vi "Import File - Rx XML.vi"(6 "Root Node":refnum<k24>, 8 "error in (no error)":errorcluster) -> (0 "error out":errorcluster, 5 "Rx Packets":T1 {"Rx Packet Data"."Endianness" items=["big-endian"=0, "little-endian"=2]})   [LabVIEW 2016, in "UDP-Custom-Device System Explorer.lvlib"]
uses:
  UDP-Custom-Device System Explorer.lvlib
  System.Xml
  Types/XML - New/ImpExp - Rx Packets Data.ctl
  <vilib>/NI Veristand/Custom Device API/Custom Device Item Info.ctl
  Types/XML - New/ImpExp - Rx Packet Data.ctl
  Shared/Types/Shared - Channel Data Type.ctl
  Shared/Types/Shared - Buffered.PacketInfo.ctl
  Shared/Types/Shared - Pointer Encoding.ctl
  <vilib>/NI VeriStand/Custom Device API/Custom Device API.lvlib
  Shared/UDP-Custom-Device Shared.lvlib
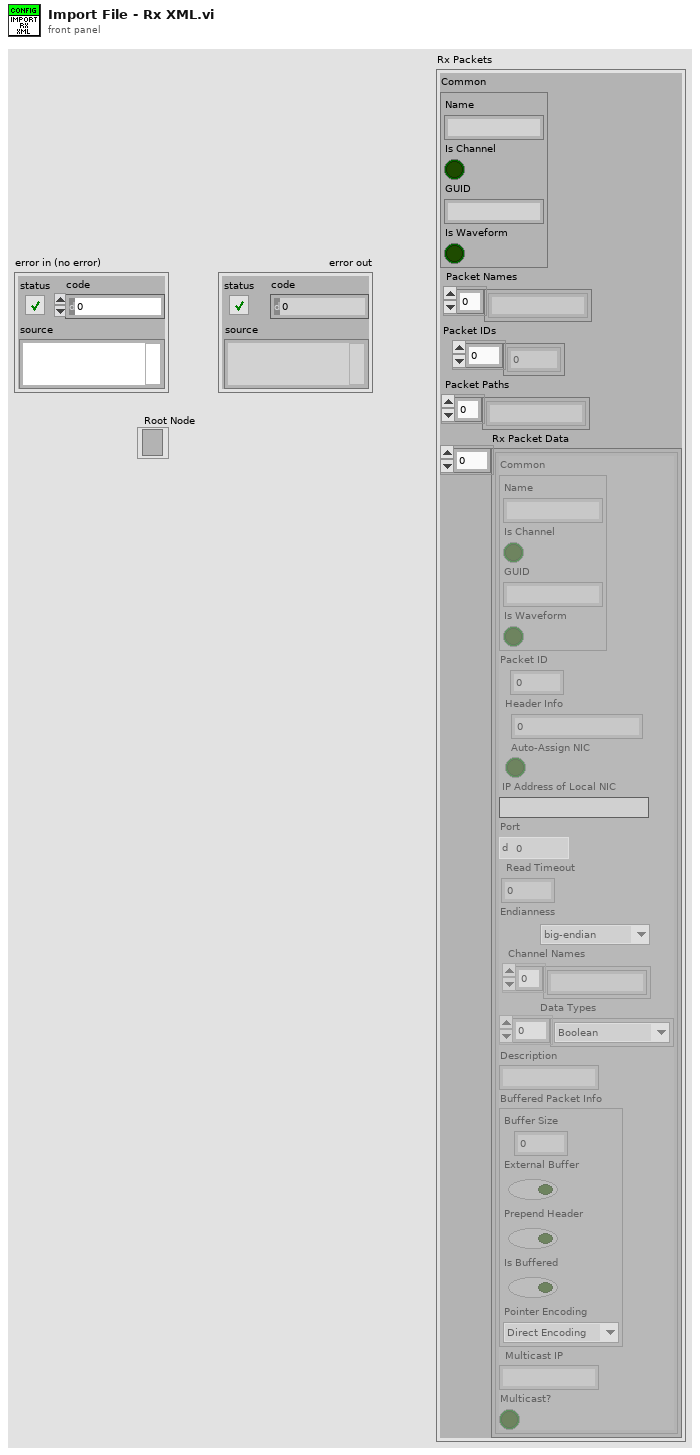
[diagram p1: front panel]
types:
  T1 = typedef "UDP-Custom-Device System Explorer.lvlib/ImpExp - Rx Packets Data.ctl" = cluster{"Common":T2, "Packet Names":string[], "Packet IDs":i32[], "Packet Paths":string[], "Rx Packet Data":T3[]}
  T2 = typedef "Custom Device API.lvlib/Custom Device Item Info.ctl" = cluster{"Name":string, "Is Channel":bool, "GUID":string, "Is Waveform":bool}
  T3 = typedef "UDP-Custom-Device System Explorer.lvlib/ImpExp - Rx Packet Data.ctl" = cluster{"Common":T2, "Packet ID":i32, "Header Info":u32, "Auto-Assign NIC":bool, "IP Address of Local NIC":string, "Port":u16, "Read Timeout":i32, "Endianness":u16, "Channel Names":string[], "Data Types":T4[], "Description":string, "Buffered Packet Info":T5, "Multicast IP":string, "Multicast?":bool}
  T4 = typedef "UDP-Custom-Device Shared.lvlib/Shared - Channel Data Type.ctl" = enum16{"Boolean", "Single", "Double", "I8", "I16", "I32", "I64", "U8", "U16", "U32", "U64"}
  T5 = typedef "UDP-Custom-Device Shared.lvlib/Shared - Buffered.PacketInfo.ctl" = cluster{"Buffer Size":i32, "External Buffer":bool, "Prepend Header":bool, "Is Buffered":bool, "Pointer Encoding":T6}
  T6 = typedef "UDP-Custom-Device Shared.lvlib/Shared - Pointer Encoding.ctl" = enum16{"Direct Encoding", "Conversion Encoding"}
  T7 = typedef "UDP-Custom-Device System Explorer.lvlib/ImpExp - Packet Headers.ctl" = cluster{"Packet Name":string, "Packet ID":string, "Packet Path":string}
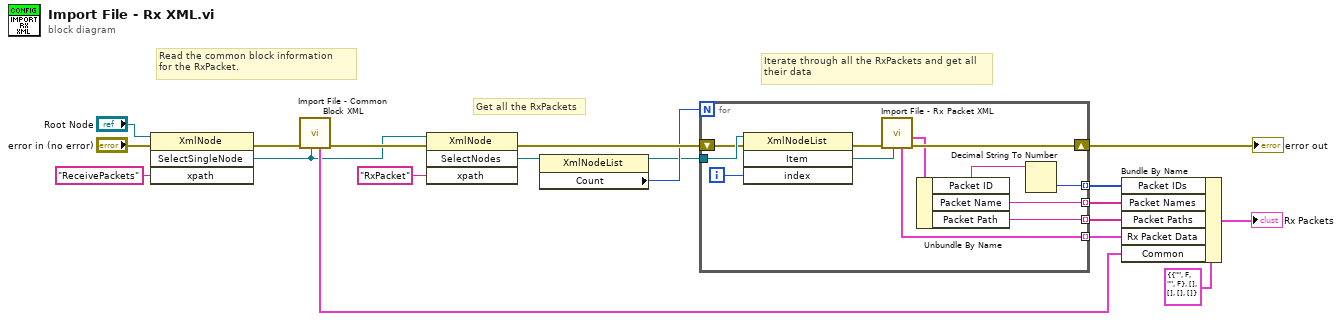
[diagram p0: block diagram]
diagram:
  # "Iterate through all the RxPackets and get all\ntheir data"
  # "Get all the RxPackets"
  # "Read the common block information\nfor the RxPacket."
  n1 = invoke class="XmlNode" method="SelectSingleNode"(reference="Root Node", error in="error in (no error)", "xpath"="ReceivePackets") -> (error out=w16:errorcluster, "SelectSingleNode"=w9:refnum<k24>)  [unwired: 1 in, 2 out]
  n2 = call "Import File - Common Block XML.vi"("Root Node"=w9, "error in (no error)"=w16) -> ("error out"=w11:errorcluster, "Common"=w14:T2)  [unwired: 8 in]
  n3 = invoke class="XmlNode" method="SelectNodes"(reference=w9, error in=w11, "xpath"="RxPacket") -> (error out=w10:errorcluster, "SelectNodes"=w7:refnum<k24>)  [unwired: 1 in, 2 out]
  n4 = property class="XmlNodeList"(reference=w7) -> (reference out=w5:refnum<k24>, "Count"=w6:i32)  [unwired: 1 in, 1 out]
  n5 = for {
    N: w6 -> [_]
    shift-right: [w27] -> w13
    shift-left: w10 -> [w30]
    tunnel: w5 -> [w31]
    tunnel: [w25] -> w4 mode=indexing
    tunnel: [w22] -> w3 mode=indexing
    tunnel: [w21] -> w2 mode=indexing
    tunnel: [w20] -> w1 mode=indexing
    i -> [w29]
    n6 = invoke class="XmlNodeList" method="Item"(reference=w31, error in=w30, "index"=w29) -> (error out=w28:errorcluster, "Item"=w26:refnum<k24>)  [unwired: 1 in, 2 out]
    n7 = call "Import File - Rx Packet XML.vi"("Root Node"=w26, "error in (no error)"=w28) -> ("error out"=w27:errorcluster, "Rx Header Data"=w24:T7, "Rx Packet"=w25:T3)  [unwired: 7 in]
    n8 = Unbundle By Name(w24) -> ("Packet ID"=w23:string, "Packet Name"=w21:string, "Packet Path"=w20:string)
    n9 = Decimal String To Number(string=w23) -> (number=w22:i32)  [unwired: 2 in, 1 out]
  }
  "error out" <- w13
  n10 = Bundle By Name(cluster=T1 {"Common"={"Name"="", "Is Channel"=FALSE, "GUID"="", "Is Waveform"=FALSE}, "Packet Names"=[], "Packet IDs"=[], "Packet Paths"=[], "Rx Packet Data"=[]} ("Rx Packets"), "Packet IDs"=w3, "Packet Names"=w2, "Packet Paths"=w1, "Rx Packet Data"=w4, "Common"=w14) -> (→"Rx Packets":T1)
